vi "WFMag_readback.vi"(10 "reference":refnum<vi>, 11 "VISA Refnum in":refnum<visa-resource-name>="COM34") -> (3 "Mag. Field (T)":string)   [LabVIEW 2014]
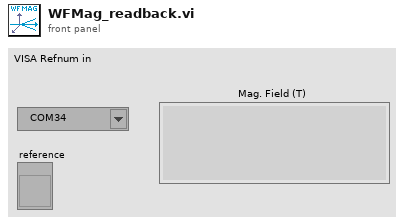
[diagram p1: front panel]
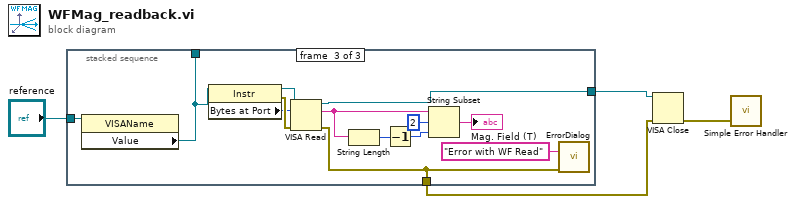
[diagram p0: block diagram]
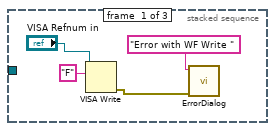
[diagram p2: hidden frame]
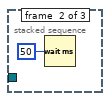
[diagram p3: hidden frame]
diagram:
  n1 = stacked-sequence {
    tunnel: [_ _ w18] -> _
    tunnel: "reference" -> [_ _ w12]
    tunnel: [_ _ w11] -> w3
    tunnel: [_ _ w10] -> w2
    frame #0 {
      n2 = VISA Write(VISA resource name="VISA Refnum in", write buffer="F") -> (error out=w6:errorcluster)  [unwired: 1 in, 2 out]
      n3 = call "ErrorDialog.vi"("error in (no error)"=w6, "message"="Error with WF Write ") -> ()  [unwired: 10 in]
    }
    frame #1 {
      n4 = Wait (ms)(milliseconds to wait=u32 50) -> ()  [unwired: 1 out]
    }
    frame #2 {
      n5 = property class="VISAName"(reference=w12) -> ("Value"=w18:refnum<visa-resource-name>)  [unwired: 1 in, 2 out]
      n6 = property class="Instr"(reference=w18) -> (reference out=w17:refnum<visa-resource-name>, error out=w16:errorcluster, "Bytes at Port"=w15:u32)  [unwired: 1 in]
      n7 = VISA Read(VISA resource name=w17, byte count=w15, error in (no error)=w16) -> (VISA resource name out=w11:refnum<visa-resource-name>, read buffer=w14:string, error out=w10:errorcluster)  [unwired: 1 out]
      n8 = String Length(string=w14) -> (length=w21:i32)
      n9 = Decrement(x=w21) -> (x-1=w20:i32)
      n10 = String Subset(string=w14, offset (0)=2 ("length (rest)"), length (rest)=w20) -> (substring=→"Mag. Field (T)":string)
      n11 = call "ErrorDialog.vi"("error in (no error)"=w10, "message"="Error with WF Read") -> ()  [unwired: 10 in]
    }
  }
  n12 = VISA Close(VISA resource name=w3, error in (no error)=w2) -> (error out=w1:errorcluster)
  n13 = call <vilib>:"Simple Error Handler.vi"("error in (no error)"=w1) -> ()  [unwired: 4 in, 5 out]
